vi "TabStyle.vi"(9 "Tab in":refnum<class "Tab.lvclass">) -> (3 "Tab out":refnum<class "Tab.lvclass">, 4 "Tab style":T1)   [LabVIEW 2014, in "Tab.lvclass"]
uses:
  Tab.lvclass
  TabStyleTD.ctl
  Control/Control.lvclass/Control.ctl
  Control/Control.lvclass
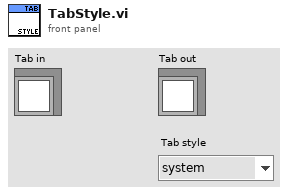
[diagram p1: front panel]
types:
  T1 = typedef "TabStyleTD.ctl" = enum16{"system", "modern", "classic"}
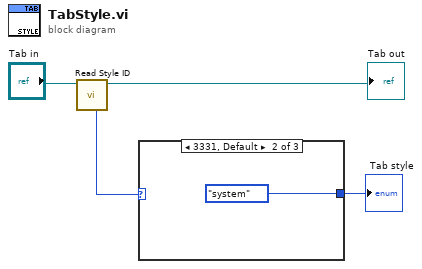
[diagram p0: block diagram]
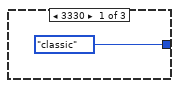
[diagram p2: hidden frame]
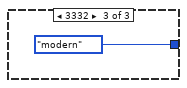
[diagram p3: hidden frame]
diagram:
  n1 = call "Read Style ID.vi"("Control in"="Tab in") -> ("Control out"=→"Tab out":refnum<class "Tab.lvclass">, "Style ID"=w2:u32)  [unwired: 7 in]
  n2 = case shown="3331, Default" w2 {
    tunnel: [TabStyleTD."classic" ("Tab index") TabStyleTD."system" ("Tab index") TabStyleTD."modern" ("Tab index")] -> w1
    frame 3330 {
    }
    frame 3331, Default {
    }
    frame 3332 {
    }
  }
  "Tab style" <- w1
